vi "MovetoNextArrayRow.vi"(8 "Error In":errorcluster, 10 "Positions":i64[](array[numeric]), 11 "MotorController in":refnum<class "MotorController.lvclass">) -> (0 "Error Out":errorcluster, 3 "MotorController out":refnum<class "MotorController.lvclass">)   [LabVIEW 2019]
uses:
  MotorController.lvclass
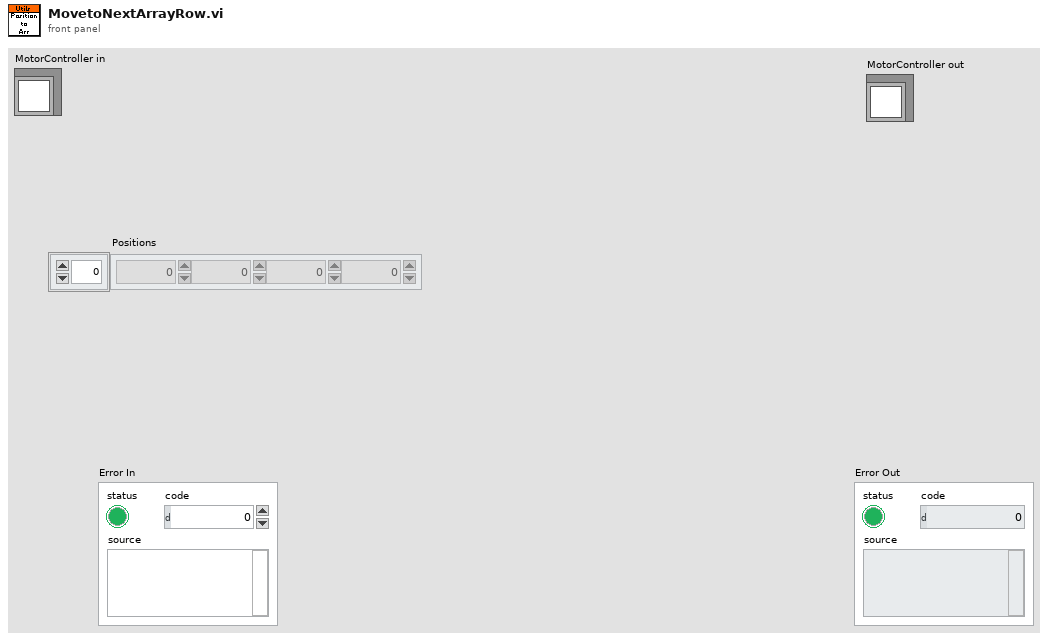
[diagram p1: front panel]
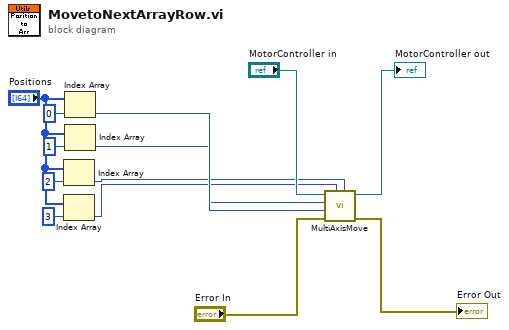
[diagram p0: block diagram]
diagram:
  n1 = Index Array(array="Positions", index=2) -> (element=w1:i64)
  n2 = Index Array(array="Positions", index=3) -> (element=w2:i64)
  n3 = Index Array(array="Positions", index=0) -> (element=w4:i64)
  n4 = Index Array(array="Positions", index=1) -> (element=w3:i64)
  n5 = call "MultiAxisMove.vi"("Polarizer 1 Position"=w1, "Polarizer 2 Position"=w2, "error in (no error)"="Error In", "Stage Position"=w4, "Sample Position"=w3, "MotorController in"="MotorController in") -> ("error out"=→"Error Out":errorcluster, "MotorController out"=→"MotorController out":refnum<class "MotorController.lvclass">)  [unwired: 4 in]
